vi "Set Transparent Color.vi"(5 "Factor":u8=255, 7 "Activate":bool=TRUE, 10 "error in (no error)":errorcluster, 11 "Color to Replace":u32(colorbox)=16777238) -> (2 "error out":errorcluster)   [LabVIEW 2014]
uses:
  User32.dll
panel:
  # "Input"
  # "Output"
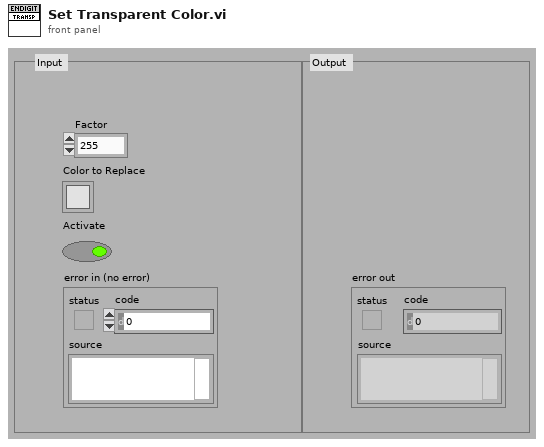
[diagram p1: front panel]
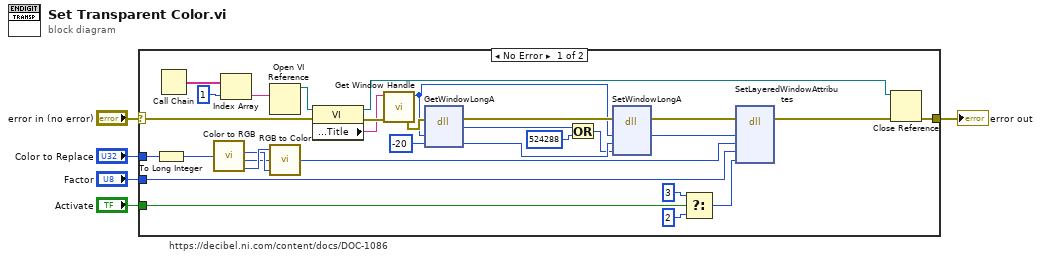
[diagram p0: block diagram]
diagram:
  # "https://decibel.ni.com/content/docs/DOC-1086"
  n1 = case shown="No Error" "error in (no error)" {
    selector: "error in (no error)" -> [w17 w37]
    tunnel: "Activate" -> [w26 _]
    tunnel: "Factor" -> [w20 _]
    tunnel: "Color to Replace" -> [w19 _]
    tunnel: [w11 w37] -> w2
    frame No Error {
      n2 = To Long Integer(number=w19) -> (32bit integer=w33:i32)
      n3 = Call Chain() -> (call chain=w14:string[])
      n4 = call <vilib>:"Color to RGB.vi"("Color"=w33) -> ("R"=w31:u8, "G"=w30:u8, "B"=w32:u8)  [unwired: 1 out]
      n5 = Index Array(array=w14, index=1) -> (element=w15:string)
      n6 = Open VI Reference(vi path=w15) -> (vi reference=w13:refnum<vi>)  [unwired: 5 in, 1 out]
      n7 = call <vilib>:"RGB to Color.vi"("B"=w31, "G"=w30, "R"=w32) -> ("Color"=w34:u32)
      n8 = property class="VI"(reference=w13, error in=w17) -> (reference out=w10:refnum<vi>, error out=w8:errorcluster, "Front Panel.Title"=w7:string)
      n9 = call "Get Window Handle.vi"("error in (no error)"=w8, "window name (\"\")"=w7) -> ("error out"=w9:errorcluster, "hWnd"=w6:u32)  [unwired: 4 in]
      n10 = dll-call lib="user32.dll" fn="GetWindowLongA" label="getWindowLong"(error in=w9, "handle"=w6, "nIndex"=-20) -> (error out=w22:errorcluster, w24:i32, "nIndex"=w36:i32)  [unwired: 3 in, 1 out]
      n11 = Or(x=w24, y=524288) -> (x .or. y?=w21:i32)
      n12 = dll-call lib="user32.dll" fn="SetWindowLongA" label="SetWindowLong"(error in=w22, "handle"=w6, "nIndex"=w36, "dwNewLong"=w21) -> (error out=w23:errorcluster, "handle"=w18:i32)  [unwired: 4 in, 2 out]
      n13 = Select(t=3, s=w26, f=2) -> (s? t:f=w27:i32)
      n14 = dll-call lib="user32.dll" fn="SetLayeredWindowAttributes" label="SetLayerdWindowAttributs"(error in=w23, "handle"=w18, "crkey"=w34, "bAlpha"=w20, "dwFlags"=w27) -> (error out=w12:errorcluster)  [unwired: 5 in, 3 out]
      n15 = Close Reference(reference=w10, error in (no error)=w12) -> (error out=w11:errorcluster)
    }
    frame Error {
    }
  }
  "error out" <- w2
